vi "Launch.vi"(11 "Response Channel":refnum<class "Messenger.lvclass">) -> (0 "error out":errorcluster)   [LabVIEW 2015, in "Main Controller Actor.lvclass"]
uses:
  Main Controller Actor.lvclass
  Re-use Libraries/Minimal Actor Framework/Messaging/Messenger/Messenger.lvclass
  Re-use Libraries/Minimal Actor Framework/Actors/Base Actor/Actor/Front Panel State.ctl
  API/Main Controller Actor API.lvclass
  Re-use Libraries/Minimal Actor Framework/Actors/Base Actor/Actor/Actor.lvclass/Actor.ctl
  Globals.vi
  Re-use Libraries/Minimal Actor Framework/Actors/Base Actor/Actor/Actor.lvclass
  Re-use Libraries/Minimal Actor Framework/Actors/Base Actor/API/Actor API.lvclass
  Re-use Libraries/Utility/Utility.lvlib
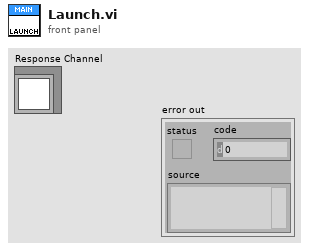
[diagram p1: front panel]
types:
  T1 = typedef "Actor.lvclass/Front Panel State.ctl" = enum32{"Invalid", "Standard", "Closed", "Hidden", "Minimized", "Maximized"}
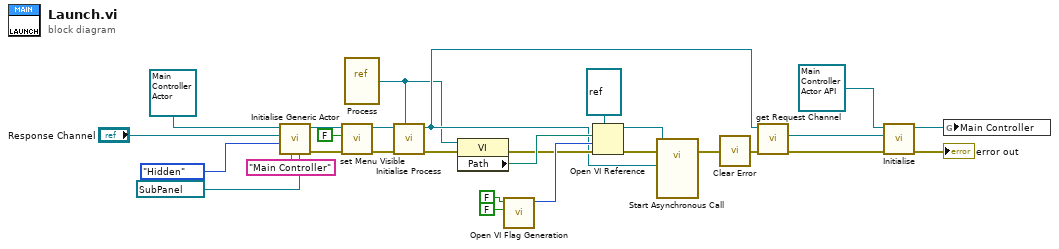
[diagram p0: block diagram]
diagram:
  n1 = call-dynamic "Initialise Generic Actor.vi"("Sub Panel"=refnum<vi> refnum, "Name"="Main Controller", "Front Panel State"=Front_Panel_State."Hidden", "Response Channel"="Response Channel", "Actor in"=refnum<class "Main Controller Actor.lvclass"> refnum ("Main Controller.lvclass")) -> ("error out"=w3:errorcluster, "Actor out"=w5:refnum<class "Main Controller Actor.lvclass">)  [unwired: 5 in]
  n2 = call "set Menu Visible.vi"("error in (no error)"=w3, "Menu Visible"=FALSE, "Actor in"=w5) -> ("error out"=w2:errorcluster, "Actor out"=w4:refnum<class "Main Controller Actor.lvclass">)  [unwired: 7 in]
  n3 = vi-ref "Process.vi"() -> (w6:refnum<vi>)
  n4 = call-dynamic "Initialise Process.vi"("Process"=w6, "error in (no error)"=w2, "Actor in"=w4) -> ("error out"=w20:errorcluster, "Actor out"=w13:refnum<class "Main Controller Actor.lvclass">)  [unwired: 7 in]
  n5 = property class="VI"(reference=w6, error in=w20) -> (error out=w21:errorcluster, "Path"=w28:path)  [unwired: 1 out]
  n6 = call "Open VI Flag Generation.vi"("Call And Collect (F)"=FALSE, "Re-entrant (F)"=FALSE) -> ("Flags"=w22:i32)  [unwired: 9 in]
  n7 = Open VI Reference(type specifier VI Refnum (for type only)=refnum<vi> refnum, vi path=w28, options=w22, error in (no error)=w21) -> (vi reference=w26:refnum<vi>, error out=w27:errorcluster)  [unwired: 2 in]
  n8 = call-by-ref "Start Asynchronous Call"(reference=w26, error in=w27, "Main Controller"=w13) -> (error out=w14:errorcluster)  [unwired: 11 in, 1 out]
  n9 = call "Clear Error.vi"("error in (no error)"=w14) -> ("error out"=w10:errorcluster)
  n10 = call "get Request Channel.vi"("error in (no error)"=w10, "Actor in"=w13) -> ("error out"=w12:errorcluster, "Request Channel"=w11:refnum<class "Messenger.lvclass">)  [unwired: 7 in, 1 out]
  n11 = call "Initialise.vi"("error in (no error)"=w12, "Request Channel"=w11, "Actor API in"=refnum<class "Main Controller Actor API.lvclass"> refnum ("Main Controller Actor API.lvclass")) -> ("error out"=→"error out":errorcluster, "Actor API out"=w8:refnum<class "Main Controller Actor API.lvclass">)  [unwired: 7 in]
  n12 = global write "Globals.vi" "Main Controller"(w8) -> ()
